vi "find flat instance.vi"(8 "error in":errorcluster, 10 "ID":string, 11 "flat hierarchy":T2) -> (0 "error out":errorcluster, 3 "instancedata":T1)   [LabVIEW 2025, in "CEF.lvlib"]
doc: "Searches a flattened instance set for the instance with a given ID.Copyright 2017 National Instruments Corporation\n\nLicensed under the Apache License, Version 2.0 (the \"License\"); you may not use this file except in compliance with the License. You may obtain a copy of the License at http://www.apache.org/licenses/LICENSE-2.0\nUnless required by applicable law or agreed to in writing, software distributed under the License is distributed on an \"AS IS\" BASIS, WITHOUT WARRANTIES OR CONDITIONS OF ANY KIND, either express or implied. See the License for the specific language governing permissions and limitations under the License."
uses:
  CEF.lvlib
  flat hierarchy.ctl
  hierarchy repo/full hierarchy.ctl
  hierarchy element.ctl
  instance data.ctl
  hierarchy repo/CEF_HierarchyRepo.lvclass
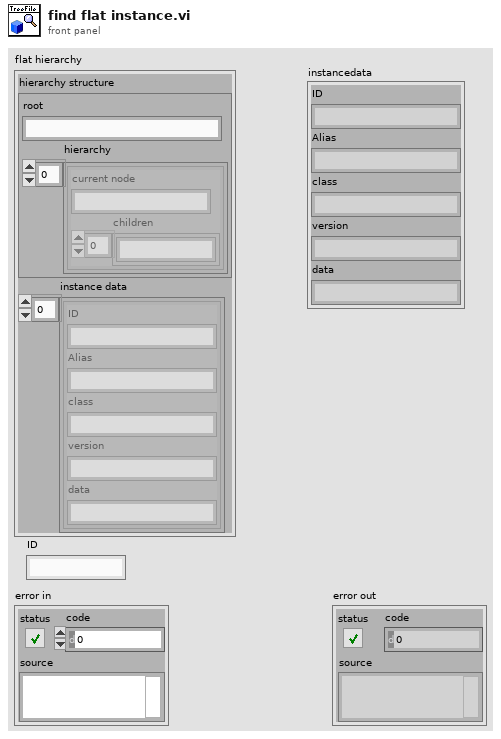
[diagram p1: front panel]
types:
  T1 = typedef "CEF.lvlib/instance data.ctl" = cluster{"ID":string, "Alias":string, "class":string, "version":string, "data":string}
  T2 = typedef "CEF.lvlib/flat hierarchy.ctl" = cluster{"hierarchy structure":T3, "instance data":T1[]}
  T3 = typedef "CEF.lvlib/CEF_HierarchyRepo.lvclass/full hierarchy.ctl" = cluster{"root":string, "hierarchy":T4[]}
  T4 = typedef "CEF.lvlib/hierarchy element.ctl" = cluster{"current node":string, "children":string[]}
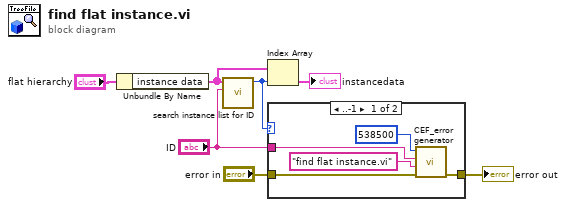
[diagram p0: block diagram]
diagram:
  n1 = Unbundle By Name("flat hierarchy") -> ("instance data"=w6:T1[])
  n2 = call "search instance list for ID.vi"("UID"="ID", "instance data"=w6) -> ("index"=w4:i32)  [unwired: 9 in]
  n3 = Index Array(array=w6, index=w4) -> (element=→"instancedata":T1)
  n4 = case shown="..-1" w4 {
    tunnel: [w11 w13] -> w3
    tunnel: "error in" -> [w12 w13]
    tunnel: "ID" -> [w9 _]
    frame ..-1 {
      n5 = call "CEF_error generator.vi"("error in"=w12, "source"="find flat instance.vi", "append error message"=w9, "error code (0)"=538500) -> ("error out"=w11:errorcluster)  [unwired: 5 in]
    }
    frame 0.. {
    }
  }
  "error out" <- w3
